vi "Get All Input Parameters.vi"(8 "error in (no error)":errorcluster, 11 "VI Call In":refnum<class "VI Server VI Call.lvclass">) -> (0 "error out":errorcluster, 2 "Input Parameters":map{string, variant}(c390))   [LabVIEW 2020, in "VI Server VI Call.lvclass"]
uses:
  VI Server VI Call.lvclass
  VI Server VI Call.lvclass/VI Server VI Call.ctl
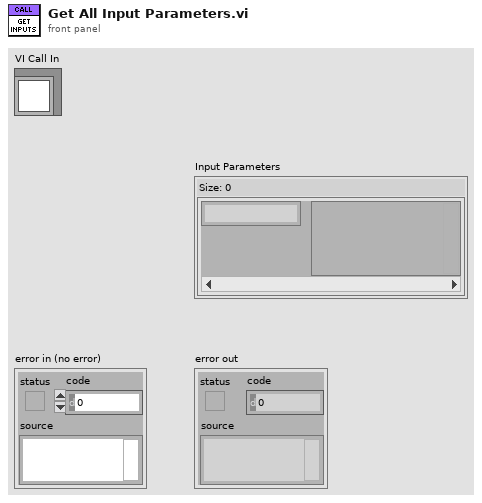
[diagram p1: front panel]
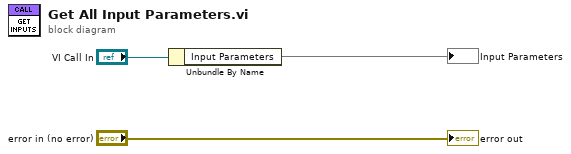
[diagram p0: block diagram]
diagram:
  n1 = Unbundle By Name("VI Call In") -> ("Input Parameters"=→"Input Parameters":map{string, variant})
  "error out" <- "error in (no error)"
